vi "IMAQ FPGA Camera Link Data to Pixels 4 Tap 8-Bit.vi"(1 "Camera Link Data":T1) -> (0 "Pixels":u8[](array[numeric]))   [LabVIEW 2020]
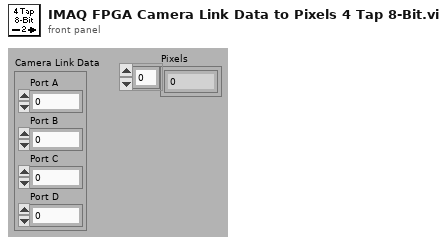
[diagram p1: front panel]
types:
  T1 = cluster{"Port A":u8, "Port B":u8, "Port C":u8, "Port D":u8}
  T2 = cluster{"Pixel 0":u8, "Pixel 1":u8, "Pixel 2":u8, "Pixel 3":u8}
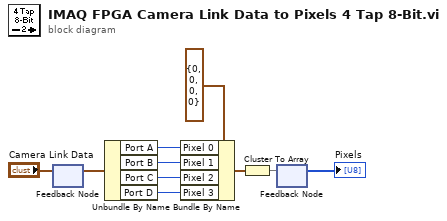
[diagram p0: block diagram]
diagram:
  n1 = feedback-in #1("Camera Link Data") -> ()
  n2 = feedback #1() -> (w3:T1)  [unwired: 1 in]
  n3 = Unbundle By Name(w3) -> ("Port A"=w8:u8, "Port B"=w7:u8, "Port C"=w6:u8, "Port D"=w5:u8)
  n4 = Bundle By Name(cluster=T2 {"Pixel 0"=0, "Pixel 1"=0, "Pixel 2"=0, "Pixel 3"=0} ("PixelData"), "Pixel 0"=w8, "Pixel 1"=w7, "Pixel 2"=w6, "Pixel 3"=w5) -> (w9:T2)
  n5 = Cluster To Array(cluster=w9) -> (array=w2:u8[])
  n6 = feedback #2() -> (→"Pixels":u8[])  [unwired: 1 in]
  n7 = feedback-in #2(w2) -> ()
